vi "Speed_Computation_2.vi"(10 "Desired position":dbl[](array[numeric]), 11 "Current position":dbl[](array[numeric])) -> (2 "Speed":dbl[](array[numeric]))   [LabVIEW 2015]
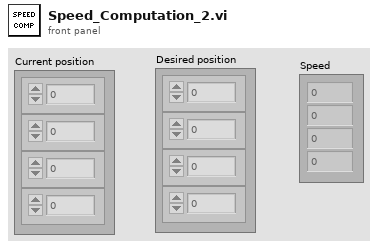
[diagram p1: front panel]
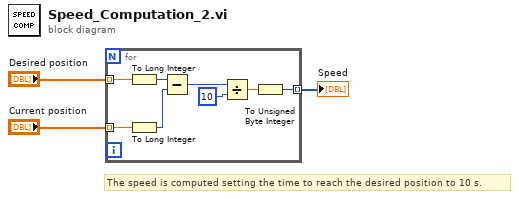
[diagram p0: block diagram]
diagram:
  # "The speed is computed setting the time to reach the desired position to 10 s."
  n1 = for {
    tunnel: "Current position" -> [w11] mode=indexing
    tunnel: "Desired position" -> [w10] mode=indexing
    tunnel: [w9] -> w1 mode=indexing
    n2 = To Long Integer(number=w10) -> (32bit integer=w6:i32)
    n3 = To Long Integer(number=w11) -> (32bit integer=w5:i32)
    n4 = Subtract(x=w6, y=w5) -> (x-y=w7:i32)
    n5 = Divide(x=w7, y=10) -> (x/y=w4:dbl)
    n6 = To Unsigned Byte Integer(number=w4) -> (unsigned 8bit integer=w9:u8)
  }
  "Speed" <- w1
